vi "AWG Make Butterfly Scripts for 1Channel.vi"(1 "Voltages":dbl[](array[numeric]), 2 "Prefix":string) -> (0 "String":string)   [LabVIEW 2013]
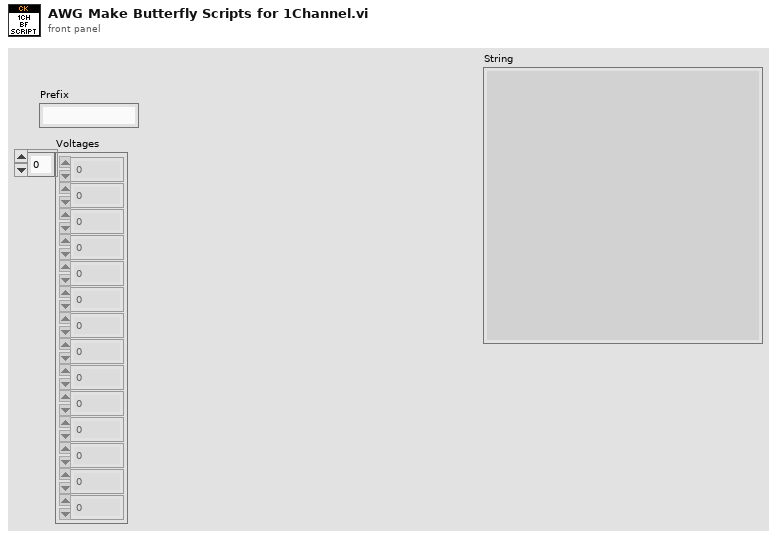
[diagram p1: front panel]
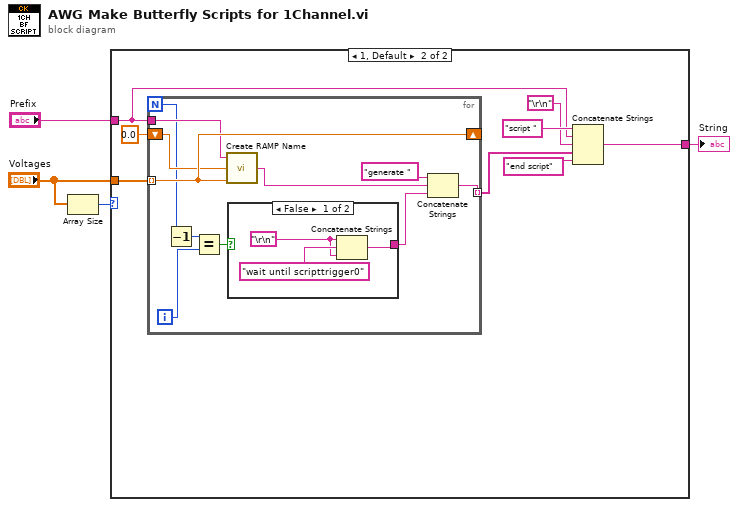
[diagram p0: block diagram]
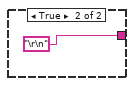
[diagram p3: hidden frame]
diagram:
  n1 = Array Size(array="Voltages") -> (size(s)=w2:i32)
  n2 = case shown="1, Default" w2 {
    tunnel: "Prefix" -> [_ w9]
    tunnel: "Voltages" -> [_ w11]
    tunnel: [_ w5] -> w1
    frame 0 {
    }
    frame 1, Default {
      n3 = for {
        N -> [w16]
        tunnel: w11 -> [w23] mode=indexing
        shift-right: [w23] -> _
        shift-left: 0.0 ("Numeric") -> [w22]
        tunnel: w9 -> [w21]
        tunnel: [w15] -> w7 mode=indexing
        i -> [w18]
        n4 = Decrement(x=w16) -> (x-1=w17:i32)
        n5 = Equal?(x=w17, y=w18) -> (x = y?=w19:bool)
        n6 = call "Create RAMP Name.vi"("Numeric 2"=w23, "Numeric 1"=w22, "Prefix"=w21) -> ("concatenated string"=w20:string)
        n7 = case shown="False" w19 {
          tunnel: [w26 "\r\n"] -> w14
          frame False {
            w24 = "\r\n"
            n8 = Concatenate Strings(w24, "wait until scripttrigger0", w24) -> (w26:string)
          }
          frame True {
          }
        }
        n9 = Concatenate Strings("generate " ("string"), w20, w14) -> (w15:string)
      }
      n10 = Concatenate Strings("script " ("string"), w9, "\r\n", w7, "end script" ("string")) -> (w5:string)
    }
  }
  "String" <- w1
